vi "ObtainProjectItems.vi"() -> ()   [LabVIEW 2016]
uses:
  TemplateLibraryItems.ctl
panel:
  out "Array 6":string[](array[string])
  out "Array 5":string[](array[string])
  out "Array 4":string[](array[string])
  out "Array 3":string[](array[string])
  out "Array 2":string[](array[string])
  out "Array":string[](array[string])
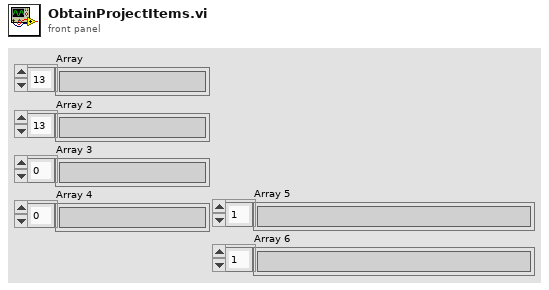
[diagram p1: front panel]
types:
  T1 = typedef "TemplateLibraryItems.ctl" = cluster{"ItemRefs":refnum<vi>[], "ItemNames":string[]}
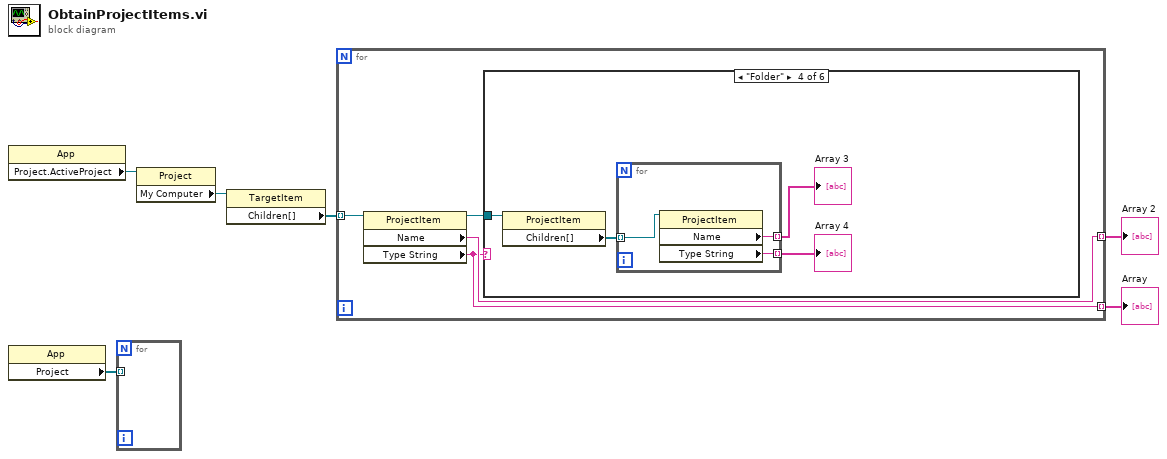
[diagram p0: block diagram]
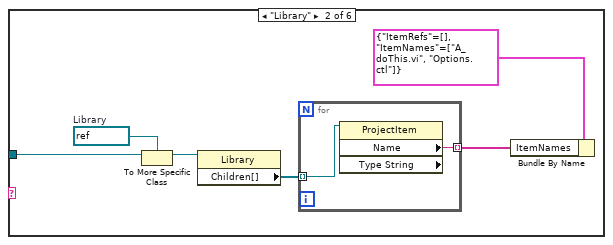
[diagram p3: hidden frame]
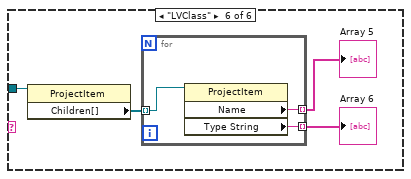
[diagram p6: hidden frame]
diagram:
  n1 = property class="App"() -> ("Project.ActiveProject"=w6:refnum<vi>)  [unwired: 2 in, 2 out]
  n2 = property class="App"() -> ("Project"=w1:refnum<vi>[])  [unwired: 2 in, 2 out]
  n3 = for {
    tunnel: w1 -> [_] mode=indexing
  }
  n4 = property class="Project"(reference=w6) -> ("My Computer"=w4:refnum<vi>)  [unwired: 1 in, 2 out]
  n5 = property class="TargetItem"(reference=w4) -> ("Children[]"=w5:refnum<vi>[])  [unwired: 1 in, 2 out]
  n6 = for {
    tunnel: w5 -> [w10] mode=indexing
    tunnel: [w9] -> w2 mode=indexing
    tunnel: [w7] -> w3 mode=indexing
    n7 = property class="ProjectItem"(reference=w10) -> (reference out=w8:refnum<vi>, "Name"=w9:string, "Type String"=w7:string)  [unwired: 1 in, 1 out]
    n8 = case shown="\"Folder\"" w7 {
      tunnel: w8 -> [_ w16 _ w22 _ w26]
      frame "False" {
      }
      frame "Library" {
        w15 = refnum<vi> refnum  # Library
        n9 = To More Specific Class(target class=w15, reference=w16) -> (specific class reference=w14:refnum<vi>)  [unwired: 1 in, 1 out]
        n10 = property class="Library"(reference=w14) -> ("Children[]"=w13:refnum<vi>[])  [unwired: 1 in, 2 out]
        n11 = for {
          tunnel: w13 -> [w18] mode=indexing
          tunnel: [w17] -> w11 mode=indexing
          n12 = property class="ProjectItem" props=["Name", "Type String"](reference=w18) -> ("Name"=w17:string)  [unwired: 1 in, 3 out]
        }
        n13 = Bundle By Name(cluster=T1 {"ItemRefs"=[], "ItemNames"=["A_doThis.vi", "Options.ctl"]} ("TemplateLibraryItems"), "ItemNames"=w11) -> ()  [unwired: 1 out]
      }
      frame "Dependencies", Default {
      }
      frame "Folder" {
        n14 = property class="ProjectItem"(reference=w22) -> ("Children[]"=w19:refnum<vi>[])  [unwired: 1 in, 2 out]
        n15 = for {
          tunnel: [w25] -> w21 mode=indexing
          tunnel: [w24] -> w20 mode=indexing
          tunnel: w19 -> [w23] mode=indexing
          n16 = property class="ProjectItem"(reference=w23) -> ("Name"=w25:string, "Type String"=w24:string)  [unwired: 1 in, 2 out]
        }
        "Array 3" <- w21
        "Array 4" <- w20
      }
      frame "VI" {
      }
      frame "LVClass" {
        n17 = property class="ProjectItem"(reference=w26) -> ("Children[]"=w27:refnum<vi>[])  [unwired: 1 in, 2 out]
        n18 = for {
          tunnel: [w32] -> w29 mode=indexing
          tunnel: [w31] -> w28 mode=indexing
          tunnel: w27 -> [w30] mode=indexing
          n19 = property class="ProjectItem"(reference=w30) -> ("Name"=w32:string, "Type String"=w31:string)  [unwired: 1 in, 2 out]
        }
        "Array 5" <- w29
        "Array 6" <- w28
      }
    }
  }
  "Array" <- w3
  "Array 2" <- w2
